vi "HEWH Extract At Index.vi"(8 "Error In":errorcluster, 10 "Test Start Index in":i32, 11 "all rows in":string[][](array[string])) -> (0 "Error Out":errorcluster, 1 "Data w/ Header":string[][](array[string]), 2 "Test Start Index out":i32, 3 "Data w/o Header":string[][](array[string]))   [LabVIEW 2019]
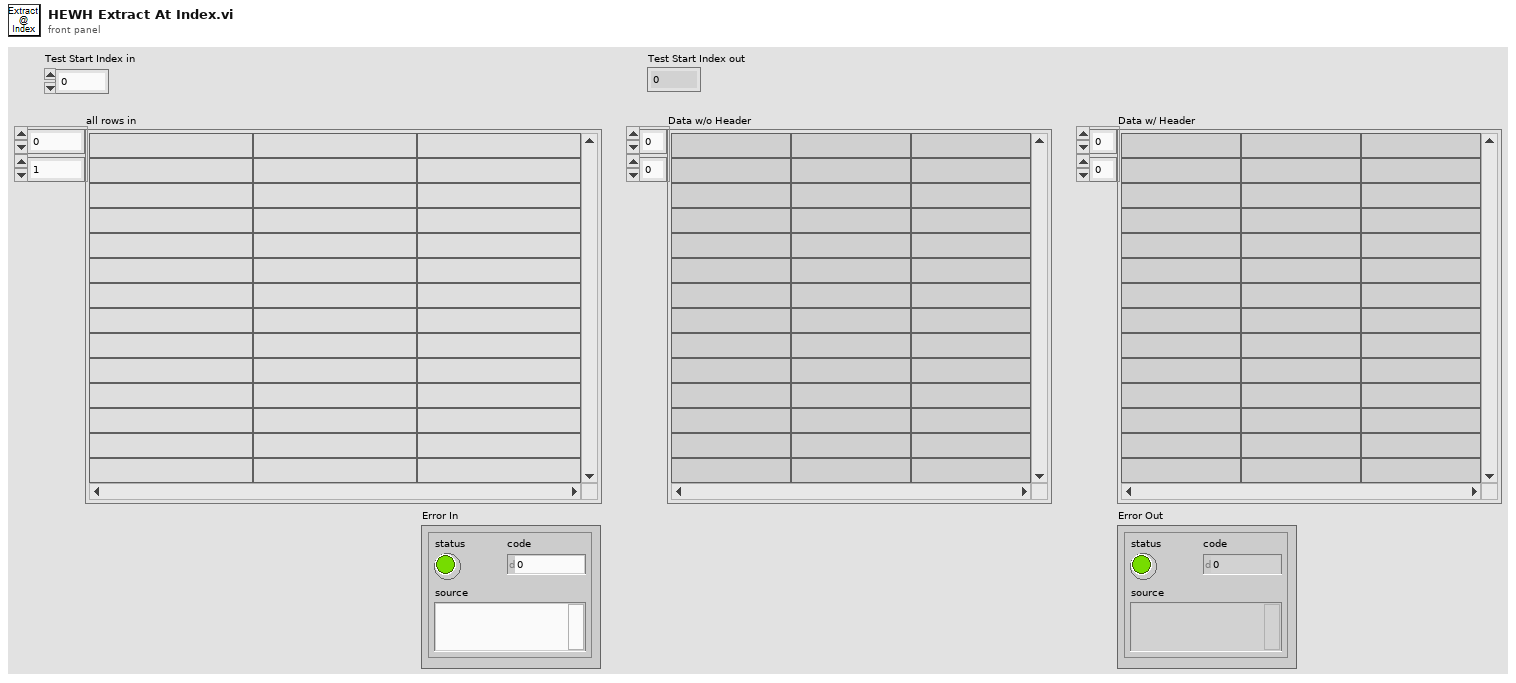
[diagram p1: front panel]
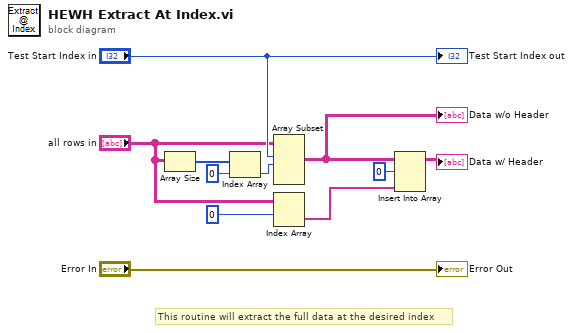
[diagram p0: block diagram]
diagram:
  # "This routine will extract the full data at the desired index"
  n1 = Array Size(array="all rows in") -> (size(s)=w8:i32[])
  n2 = Index Array(array=w8, index=0) -> (element=w10:i32)
  n3 = Array Subset(array="all rows in", index (row)="Test Start Index in", length (row)=w10) -> (w4:string[][])  [unwired: 2 in]
  "Data w/o Header" <- w4
  n4 = Index Array(array="all rows in", index (row)=0) -> (element=w3:string[])  [unwired: 1 in]
  n5 = Insert Into Array(array=w4, index (row)=0, new element=w3) -> (→"Data w/ Header":string[][])  [unwired: 1 in]
  "Test Start Index out" <- "Test Start Index in"
  "Error Out" <- "Error In"
